vi "23384_Davis_Poku_Amankwa_Amankwa.DavisPoku.MNE1201.5.4_348259_1194119229.vi"() -> ()   [LabVIEW 2018]
panel:
  in  "AM PARAMETERS":T1
  in  "Digitizing Parameters":T2
  # "a. The file size reduced by up to 5 times, and this is due to the fact that the data is now read as binary hence requires less space\n\nb.The data is well presented into to named columns, but the JK has been concatenated to the name of the first column.\n\nc. The reason why binary format has a lesser size is because while spreadsheet storage containes  several delimeters, binary storage does not\n\n\nd. By changing the value of the format constant, the size of the file chages accordinly. In order to double the size of the file we can set the value to %16.10f."
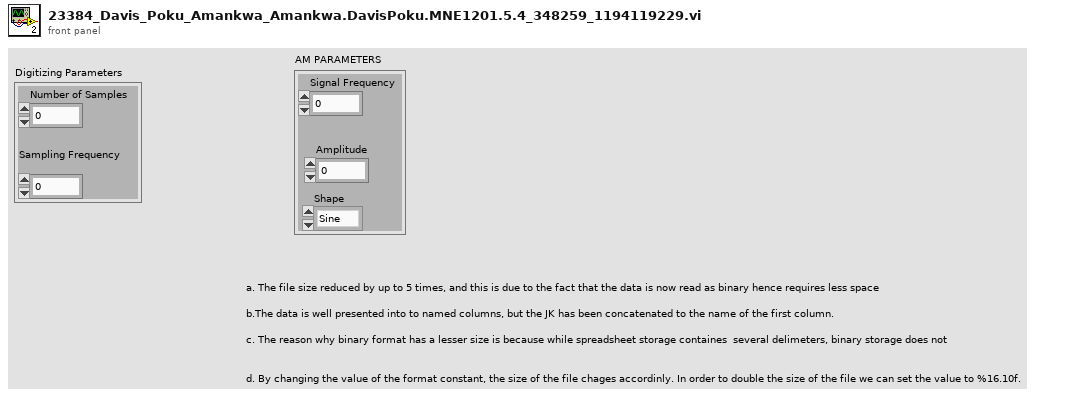
[diagram p1: front panel]
types:
  T1 = cluster{"Signal Frequency":dbl, "Amplitude":dbl, "Shape":enum16{"Sine", "Cosine", "DC Level", "Square", "User-Defined"}}
  T2 = cluster{"Number of Samples":dbl, "Sampling Frequency":dbl}
  T3 = enum16{"open", "replace", "create", "open or create", "replace or create", "replace or create with confirmation"}
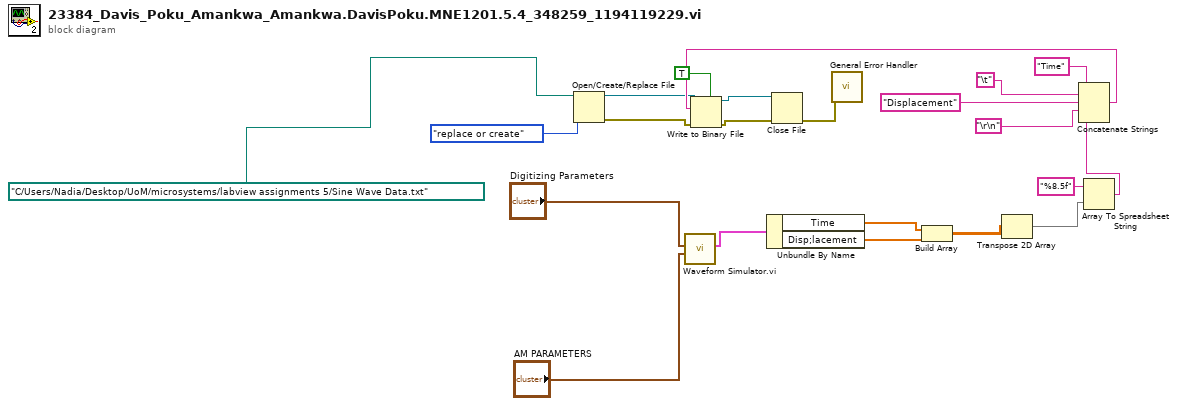
[diagram p0: block diagram]
diagram:
  n1 = Open/Create/Replace File(file path (use dialog)=path "C:/Users/Nadia/Desktop/UoM/microsystems/labview assignments 5/Sine Wave Data.txt", operation (0:open)=T3."replace or create") -> (refnum out=w5:refnum<file>, error out=w4:errorcluster)  [unwired: 4 in, 1 out]
  n2 = call "Waveform Simulator.vi.vi"("AM PARAMETERS"="AM PARAMETERS", "Digitizing Parameters"="Digitizing Parameters") -> ("Waveform Output"=w20:cluster{"Time":dbl[], "Disp;lacement":dbl[]})  [unwired: 9 in]
  n3 = Unbundle By Name(w20) -> ("Time"=w19:dbl[], "Disp;lacement"=w18:dbl[])
  n4 = Build Array(w19, w18) -> (w17:dbl[][])
  n5 = Transpose 2D Array(2D array=w17) -> (transposed array=w16:dbl[][])
  n6 = Array To Spreadsheet String(array=w16, 3:"%8.5f" ("format string")) -> (spreadsheet string=w10:string)  [unwired: 1 in]
  n7 = Concatenate Strings("Time" ("string"), "\t", "Displacement" ("string"), "\r\n", w10) -> (w9:string)
  n8 = Write to Binary File(file (use dialog)=w5, data=w9, error in=w4, 5:TRUE ("prepend array or string size? (T)")) -> (refnum out=w8:refnum<file>, error out=w7:errorcluster)  [unwired: 2 in, 1 out]
  n9 = Close File(refnum=w8, error in=w7) -> (error out=w6:errorcluster)  [unwired: 1 out]
  n10 = call <vilib>:"General Error Handler.vi"("error in (no error)"=w6) -> ()  [unwired: 10 in, 5 out]
